vi "AT_ERDS.vi"(0 "GEA2 Reference In":refnum<k24>, 5 "GEA Inputs":T3 {"Destination" format="%.0x"; "Source" format="%.0x"}, 7 "Array_Test":T2 {"Time to Wait (ms)" min=100; "ERD Number" format="%.0x"}, 11 "Error In":errorcluster) -> (4 "GEA2 Reference Out":refnum<k24>, 8 "Resultados AT Test":T1, 15 "Error Out":errorcluster)   [LabVIEW 2021]
uses:
  Common/LabVIEW GEA2 Toolkit/GEA3/type defs/Source_Destination.ctl
  D:/Common/LabVIEW GEA2 Toolkit/source/GEA3 DLL Source/GeaCommunication.dll
  Common/LabVIEW GEA2 Toolkit/source/GEA3 DLL Source/GeaCommunication.dll
  AT_Erd_Sequence.ctl
  Table_Result_AT_Test.ctl
  Common/LabVIEW GEA2 Toolkit/GEA3/type defs/Data Type.ctl
  Common/LabVIEW GEA2 Toolkit/GEA3/type defs/ERD Write Data In.ctl
  Common/LabVIEW GEA2 Toolkit/GEA3/library/GEA2_Toolkit.lvlib
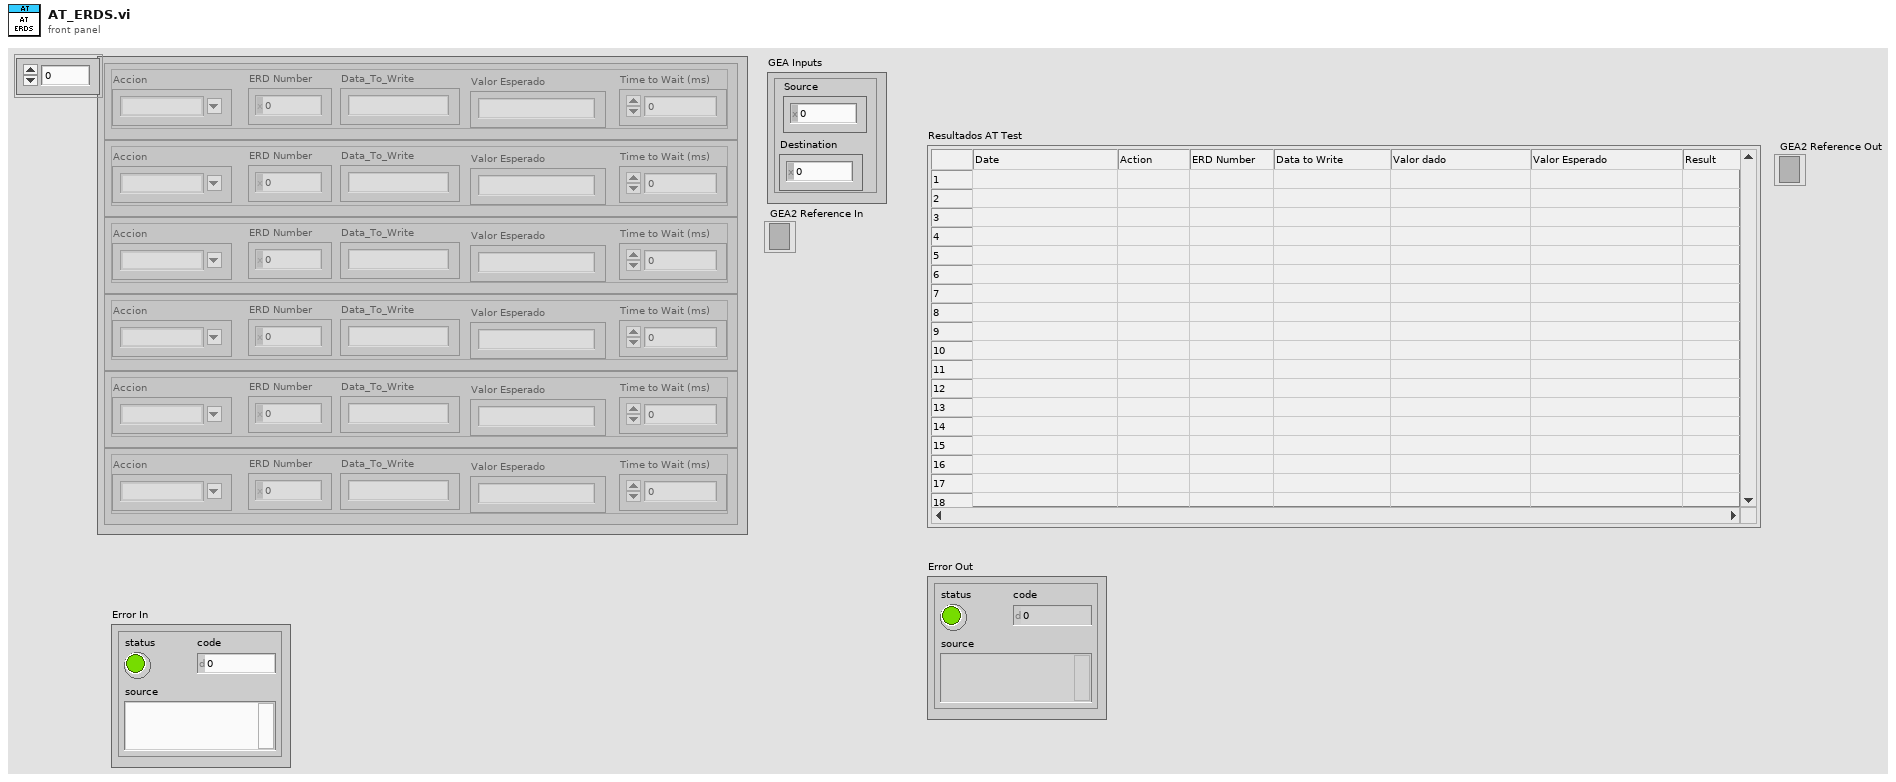
[diagram p1: front panel]
types:
  T1 = typedef "Table_Result_AT_Test.ctl" = string[][]
  T2 = typedef "AT_Erd_Sequence.ctl" = cluster{"Accion":string, "Valor Esperado":string, "ERD Number":u16, "Data_To_Write":string, "Time to Wait (ms)":u32}[]
  T3 = typedef "Source_Destination.ctl" = cluster{"Source":u8, "Destination":u8}
  T4 = typedef "Data Type.ctl" = enum16{"string", "boolean", "uint8_t", "uint16_t", "uint32_t", "uint64_t", "int8_t", "int16_t", "int32_t", "int64_t"}
  T5 = typedef "ERD Write Data In.ctl" = cluster{"ERD Number":u16, "Data Type":T4, "Data":string}
  T6 = cluster{"ERD Data Out[0]":cluster{"ERD Number":u16, "Data":string}, "ERD Data Out[1]":cluster{"ERD Number":u16, "Data":string}, "ERD Data Out[2]":cluster{"ERD Number":u16, "Data":string}, "ERD Data Out[3]":cluster{"ERD Number":u16, "Data":string}, "ERD Data Out[4]":cluster{"ERD Number":u16, "Data":string}, "ERD Data Out[5]":cluster{"ERD Number":u16, "Data":string}, "ERD Data Out[6]":cluster{"ERD Number":u16, "Data":string}, "ERD Data Out[7]":cluster{"ERD Number":u16, "Data":string}, "ERD Data Out[8]":cluster{"ERD Number":u16, "Data":string}}
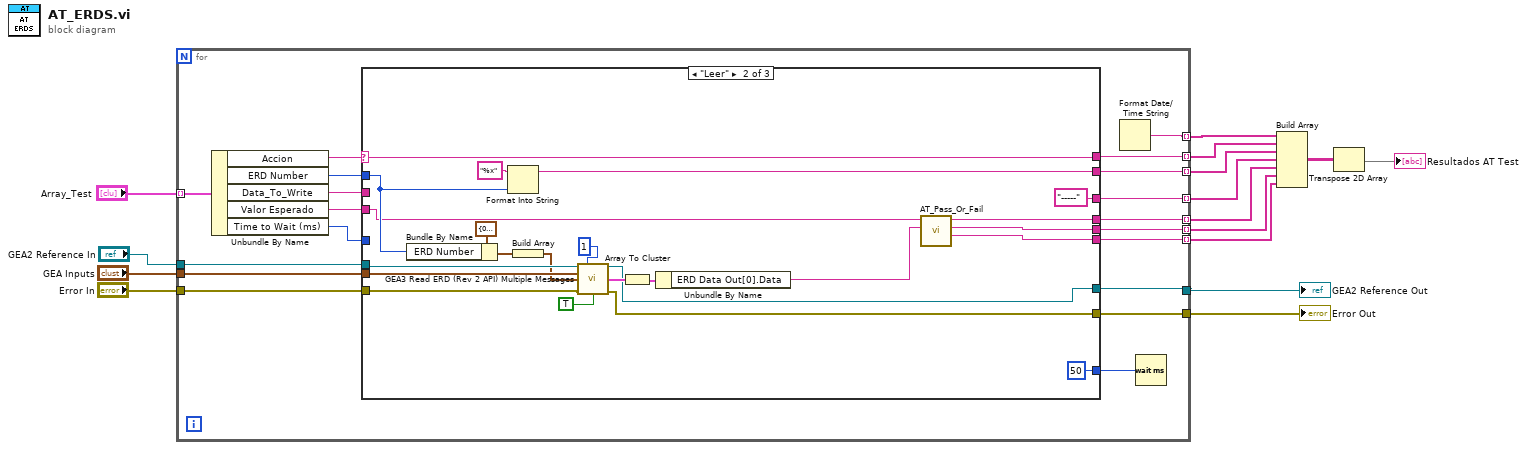
[diagram p0: block diagram]
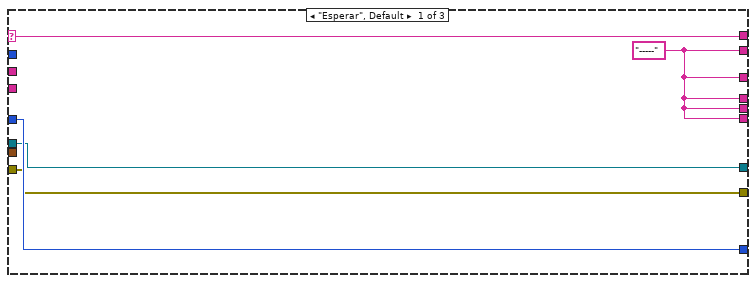
[diagram p2: hidden frame]
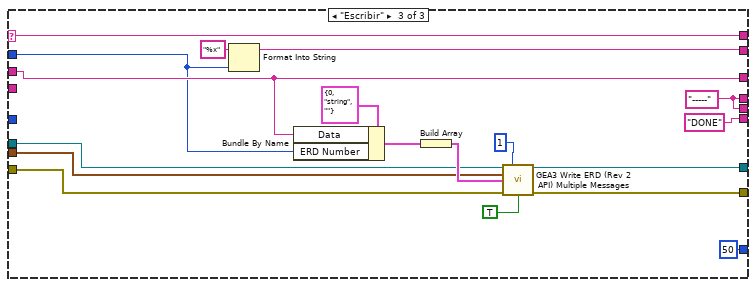
[diagram p3: hidden frame]
diagram:
  n1 = for {
    tunnel: "Array_Test" -> [w34] mode=indexing
    tunnel: [w27] -> w11 mode=indexing
    tunnel: [w26] -> w10 mode=indexing
    tunnel: [w25] -> w9 mode=indexing
    tunnel: "GEA Inputs" -> [w24]
    tunnel: "GEA2 Reference In" -> [w23]
    tunnel: "Error In" -> [w22]
    tunnel: [w21] -> w5
    tunnel: [w20] -> w4
    tunnel: [w19] -> w12 mode=indexing
    tunnel: [w18] -> w3 mode=indexing
    tunnel: [w17] -> w2 mode=indexing
    tunnel: [w16] -> w1 mode=indexing
    n2 = Unbundle By Name(w34) -> ("Accion"=w33:string, "ERD Number"=w28:u16, "Data_To_Write"=w29:string, "Valor Esperado"=w30:string, "Time to Wait (ms)"=w32:u32)
    n3 = case shown="\"Leer\"" w33 {
      selector: w33 -> [w38 w61 w79]
      tunnel: w32 -> [w39 _ _]
      tunnel: [w39 u32 50 ("Tiempo a esperar (ms)") u32 50 ("Tiempo a esperar (ms)")] -> w31
      tunnel: w30 -> [_ w43 _]
      tunnel: w29 -> [_ _ w66]
      tunnel: w28 -> [_ w48 w65]
      tunnel: [w38 w61 w79] -> w27
      tunnel: [w35 w59 w77] -> w26
      tunnel: [w35 "-----" ("f") w66] -> w25
      tunnel: w24 -> [_ w50 w70]
      tunnel: w23 -> [w37 w51 w71]
      tunnel: w22 -> [w36 w47 w69]
      tunnel: [w37 w46 w68] -> w21
      tunnel: [w36 w45 w67] -> w20
      tunnel: [w35 w42 w64] -> w18
      tunnel: [w35 w41 w64] -> w17
      tunnel: [w35 w40 "DONE" ("f")] -> w16
      frame "Esperar", Default {
        w35 = "-----" ("f")
      }
      frame "Leer" {
        n4 = Bundle By Name(cluster=cluster{"ERD Number":u16, "Data Type":T4} {"ERD Number"=0, "Data Type"=enum."string"} ("ERD Read Data In"), "ERD Number"=w48) -> (w57:cluster{"ERD Number":u16, "Data Type":T4})
        n5 = Format Into String(format string="%x", w48) -> (resulting string=w59:string)  [unwired: 2 in, 1 out]
        n6 = Build Array(w57) -> (w49:cluster{"ERD Number":u16, "Data Type":T4}[])
        n7 = call "GEA3 Read ERD (Rev 2 API) Multiple Messages.vi"("GEA2 Reference In"=w51, "Retry Count"=1, "GEA Inputs"=w50, "Read ERD List"=w49, "Error In"=w47, "Verify ERD Response?"=TRUE) -> ("GEA2 Reference Out"=w46:refnum<k24>, "ERD Data Out"=w53:cluster{"ERD Number":u16, "Data":string}[], "Error Out"=w45:errorcluster)  [unwired: 6 in, 1 out]
        n8 = Array To Cluster(array=w53) -> (cluster=w52:T6)
        n9 = Unbundle By Name(w52) -> ("ERD Data Out[0].Data"=w44:string)
        n10 = call "AT_Pass_Or_Fail.vi"("Valor Dado"=w44, "Valor Esperado"=w43) -> ("Result"=w40:string, "Valor esperado"=w41:string, "Valor dado"=w42:string)  [unwired: 7 in]
      }
      frame "Escribir" {
        w64 = "-----" ("f")
        n11 = Format Into String(format string="%x", w65) -> (resulting string=w77:string)  [unwired: 2 in, 1 out]
        n12 = Bundle By Name(cluster=T5 {"ERD Number"=0, "Data Type"=enum."string", "Data"=""} ("ERD Write Data In"), "Data"=w66, "ERD Number"=w65) -> (w73:T5)
        n13 = Build Array(w73) -> (w72:T5[])
        n14 = call "GEA3 Write ERD (Rev 2 API) Multiple Messages.vi"("GEA2 Reference In"=w71, "# of Tries"=1 ("Retry Count"), "GEA Inputs"=w70, "Write ERD List"=w72, "Error In"=w69, "Verify ERD Response?"=TRUE) -> ("GEA2 Reference Out"=w68:refnum<k24>, "Error Out"=w67:errorcluster)  [unwired: 7 in, 1 out]
      }
    }
    n15 = Format Date/Time String() -> (date/time string=w19:string)  [unwired: 3 in]
    n16 = Wait (ms)(milliseconds to wait=w31) -> ()  [unwired: 1 out]
  }
  "GEA2 Reference Out" <- w5
  "Error Out" <- w4
  n17 = Build Array(w12, w11, w10, w9, w3, w2, w1) -> (w8:string[][])
  n18 = Transpose 2D Array(2D array=w8) -> (transposed array=→"Resultados AT Test":string[][])
